vi "BS the tug main.vi"() -> ()   [LabVIEW 2012]
uses:
  <vilib>/userdefined/High Color/IMAQdx.ctl
  <vilib>/vision/driver/NI_Vision_Acquisition_Software.lvlib
  <vilib>/vision/NI_Vision_Development_Module.lvlib
panel:
  out "Scaled image":T1(plugin-control)
  out "Running?":bool
  out "All found?":bool
  in  "Data sent":string
  out "error out":errorcluster
  out "Image":T1(plugin-control)
  in  "stop":bool
  in  "Image Type":T2 items=["Grayscale (U8)", "Grayscale (I16)", "Grayscale (SGL)", "Complex (CSG)", "RGB (U32)", "HSL (U32)", "RGB (U64)", "Grayscale (U16)"]
  in  "Session In":T3="cam0"
  # "This VI receives an image from the camera above the pool and modifies the image to be 1032 x 1032 it then:\n1. Locates (4) tugs with greek letter symbols\n2. Locates (4) buoys with circle symbols\n3. Records the time the image is taken\n4. Creates a single string of that data and transmits the string using UDP to port 61557\n\nTO OPERATE START THE ROUTINE!"
  # "The Point Grey camera settings should be:\nAuto Exposure      Auto\nBrightness             Relative     200\nGain                       Auto\nFrame Rate           Absolute   20\n\nThe overhead lights should be OFF"
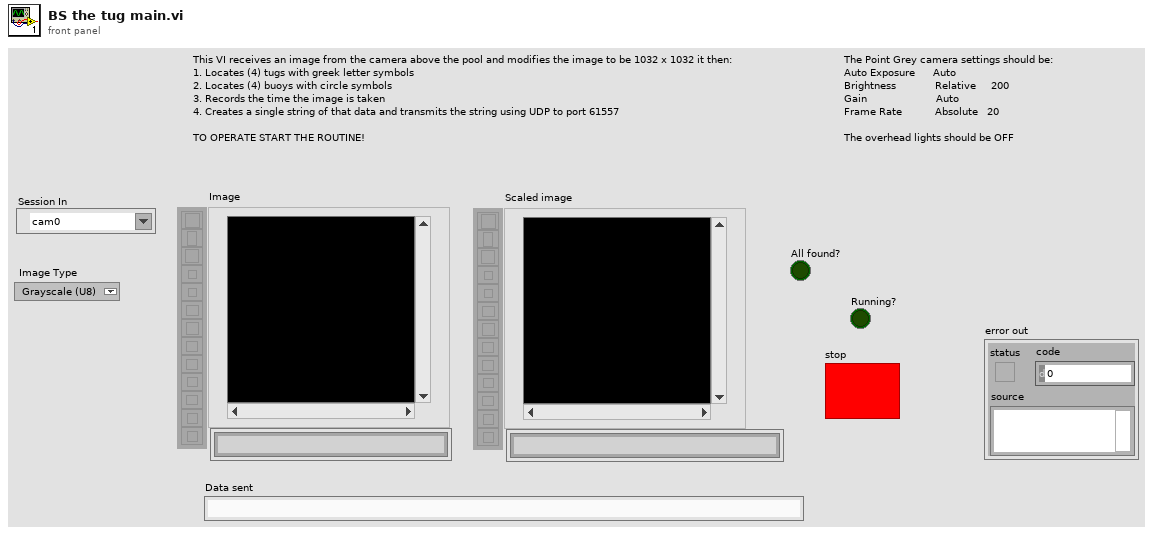
[diagram p1: front panel]
types:
  T1 = typedef "IMAQ Image.ctl" = refnum<image>
  T2 = typedef "Image Type" = u32
  T3 = typedef "IMAQdx.ctl" = refnum<k21>
  T4 = cluster{"Greek Letter":string, i16, i16, i16, bool}[]
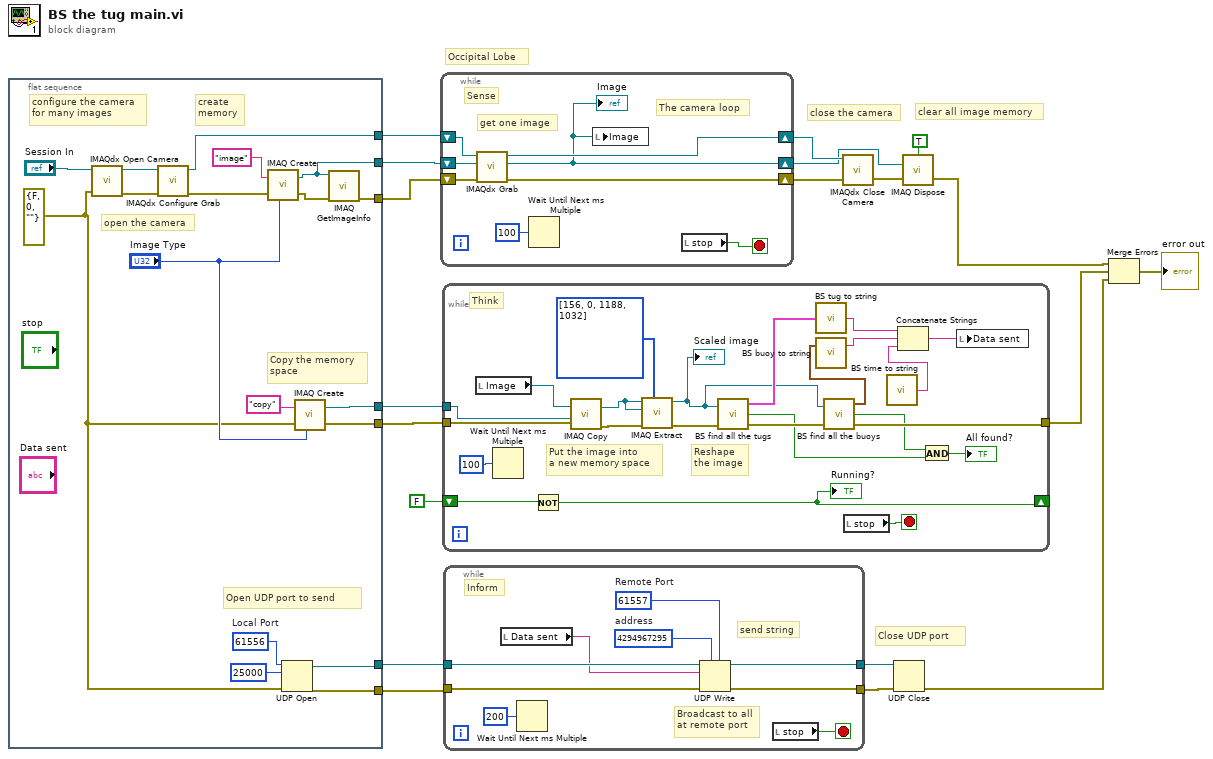
[diagram p0: block diagram]
diagram:
  # "Occipital Lobe"
  # "Close UDP port"
  # "clear all image memory"
  # "close the camera"
  n1 = flat-sequence {
    tunnel: [w31] -> w12
    tunnel: [w30] -> w13
    tunnel: [w29] -> w14
    tunnel: [w26] -> w10
    tunnel: [w25] -> w11
    tunnel: [w22] -> w4
    tunnel: [w21] -> w3
    frame #0 {
      w24 = u16 61556  # Local Port
      w20 = errorcluster {"status"=FALSE, "code"=0, "source"=""} ("error in")
      # "Open UDP port to send"
      # "Copy the memory\nspace"
      # "create\nmemory"
      # "configure the camera\nfor many images"
      # "open the camera"
      n2 = call <vilib>:"IMAQdx Open Camera.vi"("error in"=w20, "Session In"="Session In") -> ("error out"=w34:errorcluster, "Session Out"=w35:T3)  [unwired: 1 in, 7 out]
      n3 = call <vilib>:"IMAQdx Configure Grab.vi"("error in"=w34, "Session In"=w35) -> ("error out"=w36:errorcluster, "Session Out"=w30:T3)  [unwired: 8 out]
      n4 = call "IMAQ Create"("Image Name"="image", "Image Type"="Image Type", "error in (no error)"=w36) -> ("New Image"=w29:T1, "error out"=w37:errorcluster)  [unwired: 1 in, 1 out]
      n5 = UDP Open(8:w20, 9:25000 ("timeout ms (25000)"), 11:w24) -> (port=w21:refnum<k16>, 0:w22:errorcluster)  [unwired: 3 out]
      n6 = call "IMAQ Create"("Image Name"="copy", "Image Type"="Image Type", "error in (no error)"=w20) -> ("New Image"=w25:T1, "error out"=w26:errorcluster)  [unwired: 2 in]
      n7 = call "IMAQ GetImageInfo"("error in (no error)"=w37, "Image"=w29) -> ("error out"=w31:errorcluster)  [unwired: 2 in, 7 out]
    }
  }
  n8 = while {
    shift-right: [w42] -> w19
    shift-left: w13 -> [w45]
    shift-right: [w38] -> w16
    shift-left: w14 -> [w44]
    shift-right: [w41] -> w18
    shift-left: w12 -> [w43]
    stop <- w39 stop-if-true
    # "Sense"
    # "The camera loop"
    # "get one image"
    n9 = call <vilib>:"IMAQdx Grab.vi"("error in"=w43, "Image In"=w44, "Session In"=w45) -> ("error out"=w41:errorcluster, "Image Out"=w38:T1, "Session Out"=w42:T3)  [unwired: 5 in, 1 out]
    "Image" <- w38
    n10 = Wait Until Next ms Multiple(millisecond multiple=u32 100) -> ()  [unwired: 1 out]
    n11 = local write "Image"(w38) -> ()
    n12 = local read "stop"() -> (w39:bool)
  }
  n13 = while {
    tunnel: w11 -> [w64]
    tunnel: w10 -> [w65]
    tunnel: [w54] -> w8
    shift-right: [w57] -> _
    shift-left: FALSE -> [w58]
    stop <- w60 stop-if-true
    # "Think"
    # "Reshape\nthe image"
    # "Put the image into \na new memory space"
    n14 = local read "Image"() -> (w63:T1)
    n15 = Wait Until Next ms Multiple(millisecond multiple=u32 100) -> ()  [unwired: 1 out]
    n16 = Not(x=w58) -> (.not. x?=w57:bool)
    "Running?" <- w57
    n17 = call "IMAQ Copy"("error in (no error)"=w65, "Image Dst"=w64, "Image Src"=w63) -> ("error out"=w67:errorcluster, "Image Dst Out"=w68:T1)  [unwired: 3 in]
    n18 = call "IMAQ Extract"("Optional Rectangle"=i32[] [156, 0, 1188, 1032], "error in (no error)"=w67, "Image Dst"=w68, "Image Src"=w68) -> ("error out"=w62:errorcluster, "Image Dst Out"=w55:T1)  [unwired: 6 in]
    "Scaled image" <- w55
    n19 = call "BS find all the tugs.vi"("Image Src"=w55, "error in"=w62) -> ("Tug location array"=w61:T4, "All found?"=w50:bool, "error out"=w56:errorcluster)
    n20 = call "BS tug to string.vi"("Tug location array"=w61) -> ("tug location string"=w49:string)
    n21 = call "BS find all the buoys.vi"("Image Src"=w55, "error in"=w56) -> ("Buoy Array"=w52:cluster{i16, i16}[], "Buoys found?"=w51:bool, "error out"=w54:errorcluster)
    n22 = call "BS buoy to string.vi"("Buoy Array"=w52) -> ("Buoy location string"=w48:string)  [unwired: 1 in, 1 out]
    n23 = local read "stop"() -> (w60:bool)
    n24 = call "BS time to string.vi"() -> ("time string"=w47:string)  [unwired: 1 in]
    n25 = Concatenate Strings(w49, w48, w47) -> (w46:string)
    n26 = And(x=w51, y=w50) -> (x .and. y?=→"All found?":bool)
    n27 = local write "Data sent"(w46) -> ()
  }
  n28 = while {
    tunnel: w3 -> [w77]
    tunnel: w4 -> [w76]
    tunnel: [w75] -> w6
    tunnel: [w74] -> w5
    stop <- w70 stop-if-true
    w73 = u16 61557  # Remote Port
    w72 = u32 4294967295  # address
    # "Inform"
    # "send string"
    # "Broadcast to all\nat remote port"
    n29 = local read "Data sent"() -> (w71:string)
    n30 = Wait Until Next ms Multiple(millisecond multiple=u32 200) -> ()  [unwired: 1 out]
    n31 = UDP Write(address=w72, port or service name=w73, connection ID=w77, data in=w71, 8:w76) -> (error out=w75:errorcluster, 3:w74:refnum<k16>)  [unwired: 1 out]
    n32 = local read "stop"() -> (w70:bool)
  }
  n33 = call <vilib>:"IMAQdx Close Camera.vi"("error in"=w18, "Session In"=w19) -> ("error out"=w17:errorcluster)  [unwired: 9 out]
  n34 = UDP Close(connection ID=w5, 8:w6) -> (error out=w2:errorcluster)  [unwired: 1 out]
  n35 = call "IMAQ Dispose"("All Images? (No)"=TRUE, "Image"=w16, "error in (no error)"=w17) -> ("error out"=w9:errorcluster)  [unwired: 3 out]
  n36 = Merge Errors(w9, w8, w2) -> (→"error out":errorcluster)
